vi "Get Available Sets.vi"(8 "error in (no error)":errorcluster, 10 "Item Types (all visible)":T1 items=["all visible", "all including hidden", "standard only", "startup only"], 11 "Session in":refnum<k21>) -> (0 "error out":errorcluster, 2 "Software Sets":T2[](array[typedef]) {"information"."component type" items=["standard", "hidden", "system", "unknown", "startup", "image"]; "items"."component type" items=["standard", "hidden", "system", "unknown", "startup", "image"]; "add-ons"."component type" items=["standard", "hidden", "system", "unknown", "startup", "image"]}, 3 "Session out":refnum<k21>)   [LabVIEW 2014, in "nisyscfg.lvlib"]
doc: "Retrieves a list of software sets on the local system that are available for installation to the specified target. Not all Real-Time systems support the installation of software sets."
uses:
  nisyscfg.lvlib
  Software Set 1.2.ctl
  Software 1.2.ctl
  Component Type.ctl
  Component Types.ctl
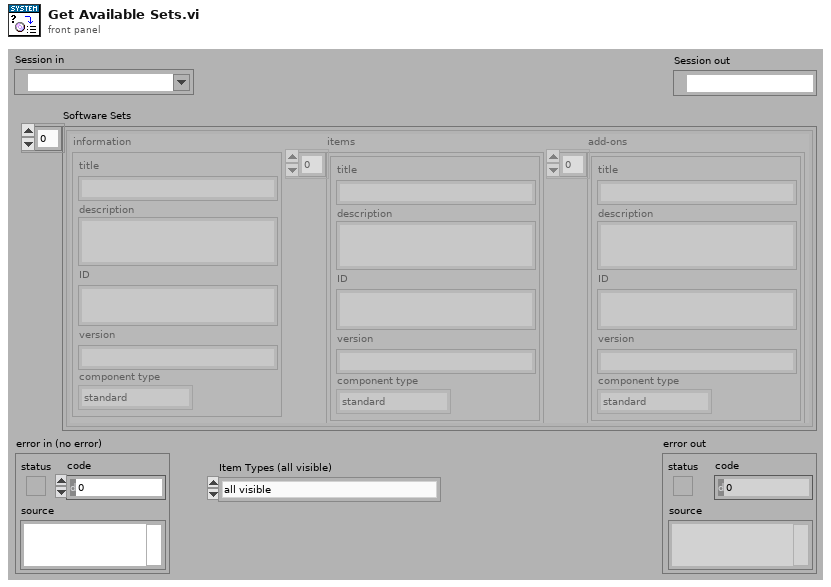
[diagram p1: front panel]
types:
  T1 = typedef "nisyscfg.lvlib/Component Types.ctl" = u32
  T2 = typedef "nisyscfg.lvlib/Software Set 1.2.ctl" = cluster{"information":T3, "items":T3[], "add-ons":T3[]}
  T3 = typedef "nisyscfg.lvlib/Software 1.2.ctl" = cluster{"title":string, "description":string, "ID":string, "version":string, "component type":T4}
  T4 = typedef "nisyscfg.lvlib/Component Type.ctl" = u32
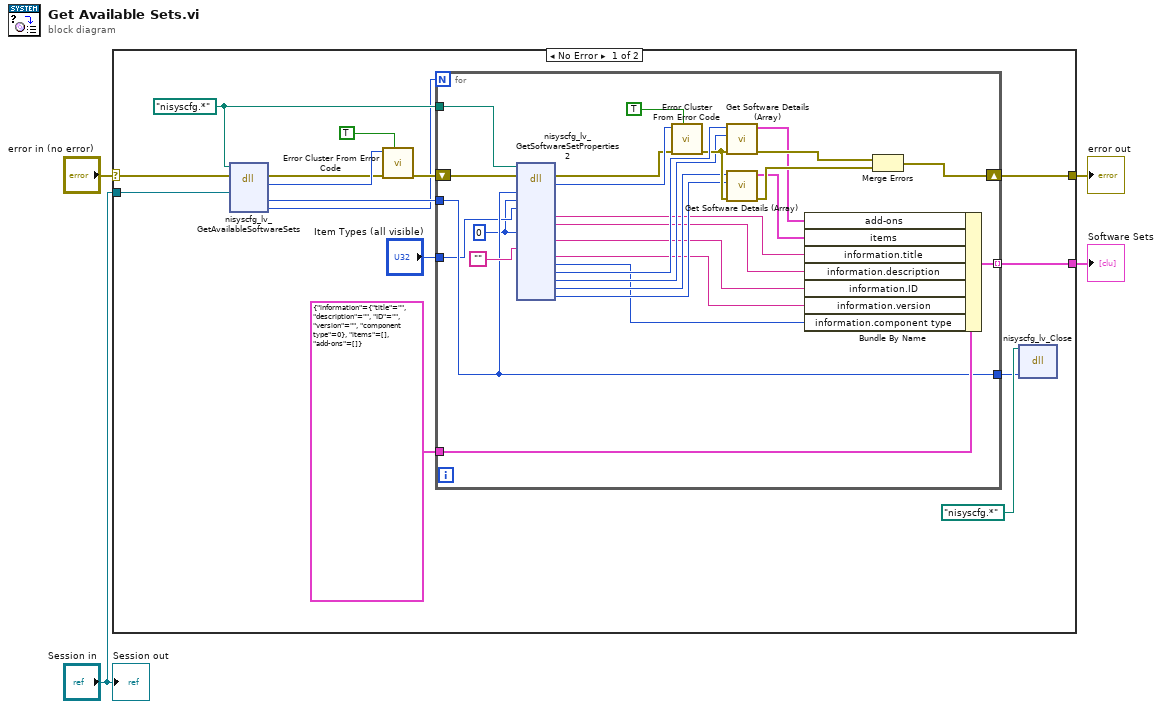
[diagram p0: block diagram]
diagram:
  n1 = case shown="No Error" "error in (no error)" {
    selector: "error in (no error)" -> [w12 w46]
    tunnel: [w15 w46] -> w4
    tunnel: "Session in" -> [w11 _]
    tunnel: [w13 _] -> w2
    frame No Error {
      w10 = path "nisyscfg.*" ("path in")
      n2 = dll-call lib="nisyscfg.*" fn="nisyscfg_lv_GetAvailableSoftwareSets" label="GetAvailableSoftwareSets"(path in=w10, error in=w12, "system"=w11) -> (error out=w17:errorcluster, "result"=w18:i32, "softwareSets"=w19:u64, "numSets"=w8:i32)  [unwired: 4 in, 1 out]
      n3 = call "Error Cluster From Error Code.vi"("show call chain? (False)"=TRUE, "error in (no error)"=w17, "error code (0)"=w18) -> ("error out"=w16:errorcluster)  [unwired: 6 in]
      n4 = for {
        N: w8 -> [_]
        tunnel: w19 -> [w31]
        shift-right: [w42] -> w15
        shift-left: w16 -> [w45]
        tunnel: T2 {"information"={"title"="", "description"="", "ID"="", "version"="", "component type"=0}, "items"=[], "add-ons"=[]} ("software set") -> [w41]
        tunnel: [w40] -> w13 mode=indexing
        tunnel: w10 -> [w39]
        tunnel: [w31] -> w6
        tunnel: "Item Types (all visible)" -> [w24]
        w23 = u8 0 ("includeAddOnDeps")
        n5 = dll-call lib="nisyscfg.*" fn="nisyscfg_lv_GetSoftwareSetProperties2" label="GetSoftwareSetProperties"(path in=w39, error in=w45, "setEnumerator"=w31, "includeAddOnDeps"=w23, "includeTypes"=w24, "type"=w23, "groupID"="") -> (error out=w43:errorcluster, "result"=w44:i32, "title"=w25:string, "description"=w26:string, "ID"=w22:string, "version"=w21:string, "visibleType"=w20:i32, "addons"=w36:u64, "numAddons"=w30:i32, "items"=w34:u64, "numItems"=w29:i32)  [unwired: 15 in, 1 out]
        n6 = call "Error Cluster From Error Code.vi"("show call chain? (False)"=TRUE, "error in (no error)"=w43, "error code (0)"=w44) -> ("error out"=w35:errorcluster)  [unwired: 6 in]
        n7 = call "Get Software Details (Array).vi"("error in (no error)"=w35, "Number of Elements"=w30, "Enumerator in"=w36) -> ("error out"=w33:errorcluster, "Software Components"=w28:T3[])  [unwired: 7 in]
        n8 = call "Get Software Details (Array).vi"("error in (no error)"=w35, "Number of Elements"=w29, "Enumerator in"=w34) -> ("error out"=w32:errorcluster, "Software Components"=w27:T3[])  [unwired: 7 in]
        n9 = Bundle By Name(cluster=w41, "add-ons"=w28, "items"=w27, "information.title"=w25, "information.description"=w26, "information.ID"=w22, "information.version"=w21, "information.component type"=w20) -> (w40:T2)
        n10 = Merge Errors(w33, w32) -> (w42:errorcluster)
      }
      n11 = dll-call lib="nisyscfg.*" fn="nisyscfg_lv_Close" label="Close"(path in=path "nisyscfg.*", "expertsEnum"=w6) -> ()  [unwired: 3 in, 3 out]
    }
    frame Error {
    }
  }
  "error out" <- w4
  "Software Sets" <- w2
  "Session out" <- "Session in"
